vi "Invoke RT VI.vi"(8 "error in (no error)":errorcluster, 9 "configuration file path":path, 10 "target alias":string, 11 "reference":refnum<vi>) -> (0 "error out":errorcluster, 1 "engine status":string, 2 "invoked VI error out":errorcluster, 3 "reference out":refnum<vi>, 5 "pass":bool)   [LabVIEW 2014]
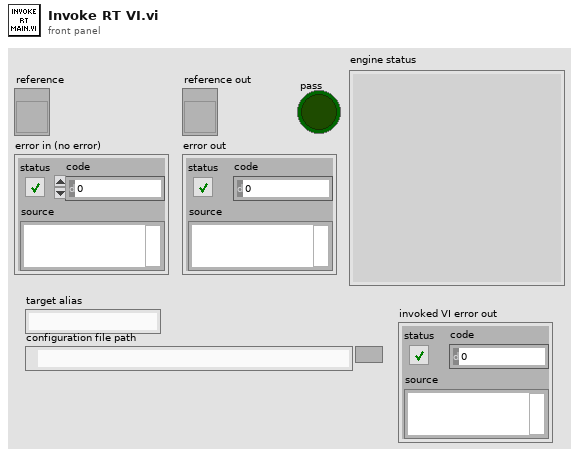
[diagram p1: front panel]
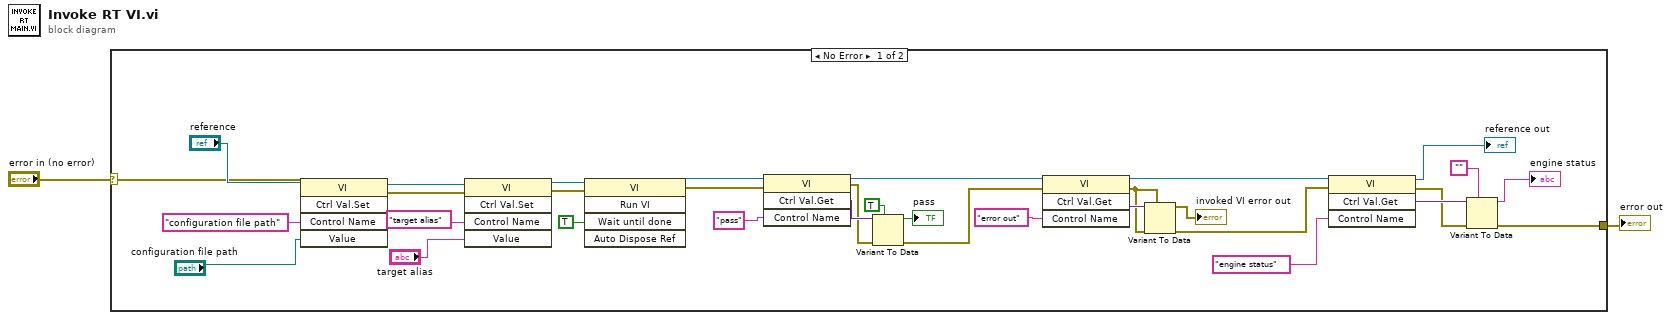
[diagram p0: block diagram]
diagram:
  n1 = case shown="No Error" "error in (no error)" {
    selector: "error in (no error)" -> [w24 w36]
    tunnel: [w14 w36] -> w2
    frame No Error {
      n2 = invoke class="VI" method="Ctrl Val.Set"(reference="reference", error in=w24, "Control Name"="configuration file path", "Value"="configuration file path") -> (reference out=w26:refnum<vi>, error out=w32:errorcluster)  [unwired: 1 in, 3 out]
      n3 = invoke class="VI" method="Ctrl Val.Set"(reference=w26, error in=w32, "Control Name"="target alias", "Value"="target alias") -> (reference out=w3:refnum<vi>, error out=w13:errorcluster)  [unwired: 1 in, 3 out]
      n4 = invoke class="VI" method="Run VI"(reference=w3, error in=w13, "Wait until done"=TRUE ("Wait Until Done")) -> (reference out=w9:refnum<vi>, error out=w10:errorcluster)  [unwired: 2 in, 3 out]
      n5 = invoke class="VI" method="Ctrl Val.Get"(reference=w9, error in=w10, "Control Name"="pass") -> (reference out=w11:refnum<vi>, error out=w6:errorcluster, "Get Control Value Variant"=w8:variant)  [unwired: 1 in, 1 out]
      n6 = Variant To Data(error in=w6, type=TRUE ("Wait Until Done"), Variant=w8) -> (data=→"pass":bool, error out=w5:errorcluster)
      n7 = invoke class="VI" method="Ctrl Val.Get"(reference=w11, error in=w5, "Control Name"="error out") -> (reference out=w23:refnum<vi>, error out=w22:errorcluster, "Get Control Value Variant"=w34:variant)  [unwired: 1 in, 1 out]
      n8 = Variant To Data(error in=w22, type=w22, Variant=w34) -> (data=→"invoked VI error out":errorcluster, error out=w21:errorcluster)
      n9 = invoke class="VI" method="Ctrl Val.Get"(reference=w23, error in=w21, "Control Name"="engine status") -> (reference out=→"reference out":refnum<vi>, error out=w15:errorcluster, "Get Control Value Variant"=w16:variant)  [unwired: 1 in, 1 out]
      n10 = Variant To Data(error in=w15, type="", Variant=w16) -> (data=→"engine status":string, error out=w14:errorcluster)
    }
    frame Error {
    }
  }
  "error out" <- w2
